vi "take_simple_data.vi"(0 "input cluster":T1) -> (5 "number of samples":i32, 7 "data tasks":T2, 10 "Actual Sample Rate":dbl=10000.0 format="%0.2f")   [LabVIEW 2018]
uses:
  <vilib>/DAQmx/create/channels.llb/DAQmx Create Channel (AI-Voltage-Basic).vi
  <vilib>/DAQmx/configure/timing.llb/DAQmx Timing (Sample Clock).vi
  <resource>/objmgr/daqmx.rc
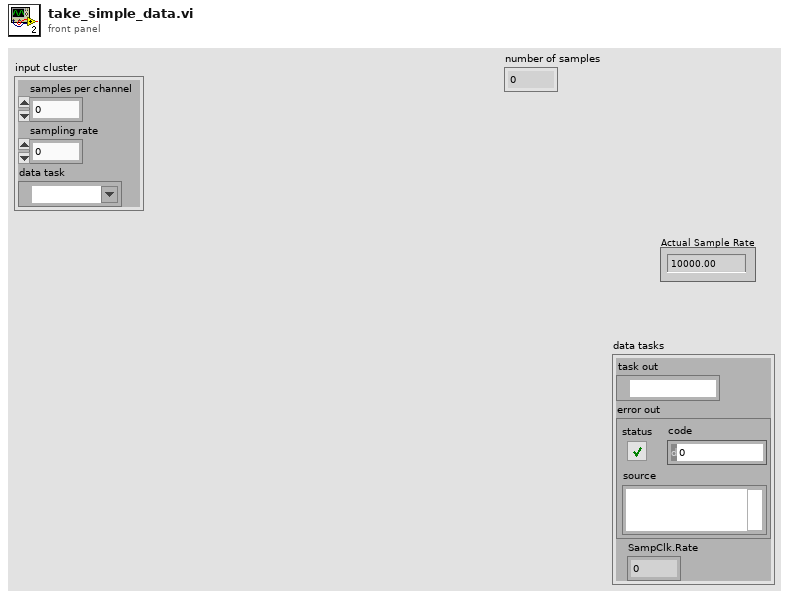
[diagram p1: front panel]
types:
  T1 = cluster{"samples per channel":dbl, "sampling rate":dbl, "data task":tag}
  T2 = cluster{"task out":refnum<k21>, "error out":errorcluster, "SampClk.Rate":dbl}
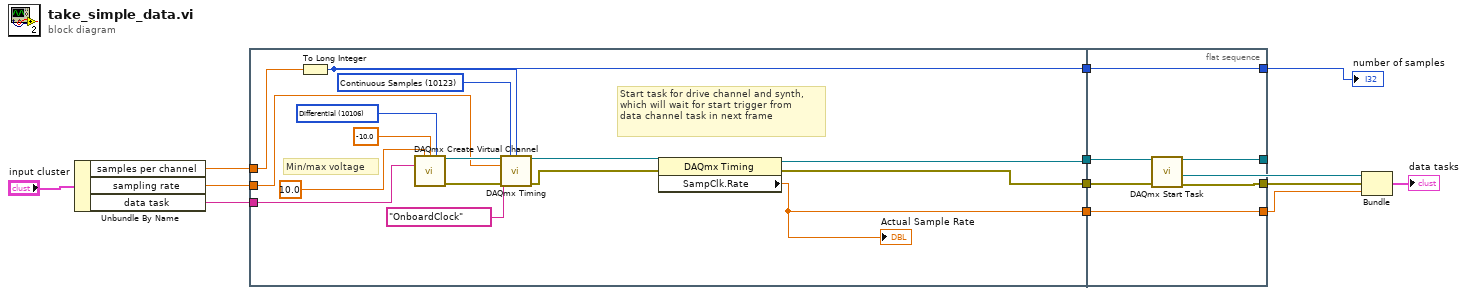
[diagram p0: block diagram]
diagram:
  n1 = Unbundle By Name("input cluster") -> ("samples per channel"=w8:dbl, "sampling rate"=w7:dbl, "data task"=w6:tag)
  n2 = flat-sequence {
    tunnel: w6 -> [w26]
    tunnel: w7 -> [w21]
    tunnel: w8 -> [w22]
    tunnel: [w18] -> w4
    tunnel: [w15] -> w3
    tunnel: [w16] -> w2
    tunnel: [w14] -> w1
    tunnel: [w34] -> w5
    tunnel: [w30] -> w12
    tunnel: [w35] -> w11
    tunnel: [w32] -> w13
    tunnel: w4 -> [w33]
    tunnel: w3 -> [w35]
    tunnel: w2 -> [w31]
    tunnel: w1 -> [w34]
    frame #0 {
      w27 = 10106 items=["default"=-1, "RSE"=10083, "NRSE"=10078, "Differential"=10106, "Pseudodifferential"=12529] ("input terminal configuration")
      w23 = 10123 items=["Finite Samples"=10178, "Continuous Samples"=10123, "Hardware Timed Single Point"=12522] ("sample mode")
      # "Start task for drive channel and synth,\nwhich will wait for start trigger from \ndata channel task in next frame"
      # "Min/max voltage"
      n3 = To Long Integer(number=w22) -> (32bit integer=w14:i32)
      n4 = call-poly <vilib>:"DAQmx Create Virtual Channel.vi"("maximum value"=10.0, "minimum value"=-10.0, "input terminal configuration"=w27, "physical channels"=w26) -> ("task out"=w28:refnum<k21>, "error out"=w29:errorcluster)  [unwired: 10 in]
      n5 = call-poly <vilib>:"DAQmx Timing.vi"("task/channels in"=w28, "sample mode"=w23, "samples per channel"=w14, "rate"=w21, "source"=tag "OnboardClock", "error in"=w29) -> ("task out"=w19:refnum<k21>, "error out"=w17:errorcluster)  [unwired: 8 in]
      n6 = property class="DAQmx Timing"(reference=w19, error in=w17) -> (reference out=w18:refnum<k21>, error out=w16:errorcluster, "SampClk.Rate"=w15:dbl)
      "Actual Sample Rate" <- w15
    }
    frame #1 {
      n7 = call <vilib>:"DAQmx Start Task.vi"("task/channels in"=w33, "error in"=w31) -> ("task out"=w32:refnum<k21>, "error out"=w30:errorcluster)  [unwired: 12 in]
    }
  }
  n8 = Bundle("task out"=w13, "error out"=w12, "SampClk.Rate"=w11) -> (→"data tasks":T2)  [unwired: 1 in]
  "number of samples" <- w5
